vi "Extract_ROIs_miniScans.vi"(8 "error in (no error)":errorcluster, 10 "ROI Attributes":T1[](array[typedef]) {"ROI group ID" format="%#_6f"; "Laser Power (%)" format="%#_6f"; "Zoom" format="%#_6f"; "Frame Size" format="%#_6f"; "Number of lines" format="%#_6f"; "Composite ID" format="%#_6f"; "Angle (deg)" format="%#_6f"; "ROI Time (ns)" format="%#_6f"; "ROI ID" format="%#_6f"; "Pixels in ROI" format="%#_6f"; "ROI index" format="%#_6f"; "Z stop" format="%#_6f"; "Y stop" format="%#_6f"; "X stop" format="%#_6f"; "Z start" format="%#_6f"; "X start" format="%#_6f"; "Y start" format="%#_6f"}) -> (0 "error out":errorcluster, 1 "Total number of miniscans":i32, 2 "miniScan_Indices":dbl[](array[numeric]), 3 "ROI Coordinates (broken down to miniscans)":T2, 4 "Zoom":dbl[](array[numeric]), 5 "Number of pixels in single X miniscan":i32, 6 "number of rectangles":i32, 7 "number of POI":i32)   [LabVIEW 2017]
uses:
  Typedefs/ROI XY coordinates cluster.ctl
  User Interface/Visualisation/Functional Imaging Viewer/Typedefs/ROI parameters data type.ctl
panel:
  out "POI_Indices":dbl[](array[numeric])
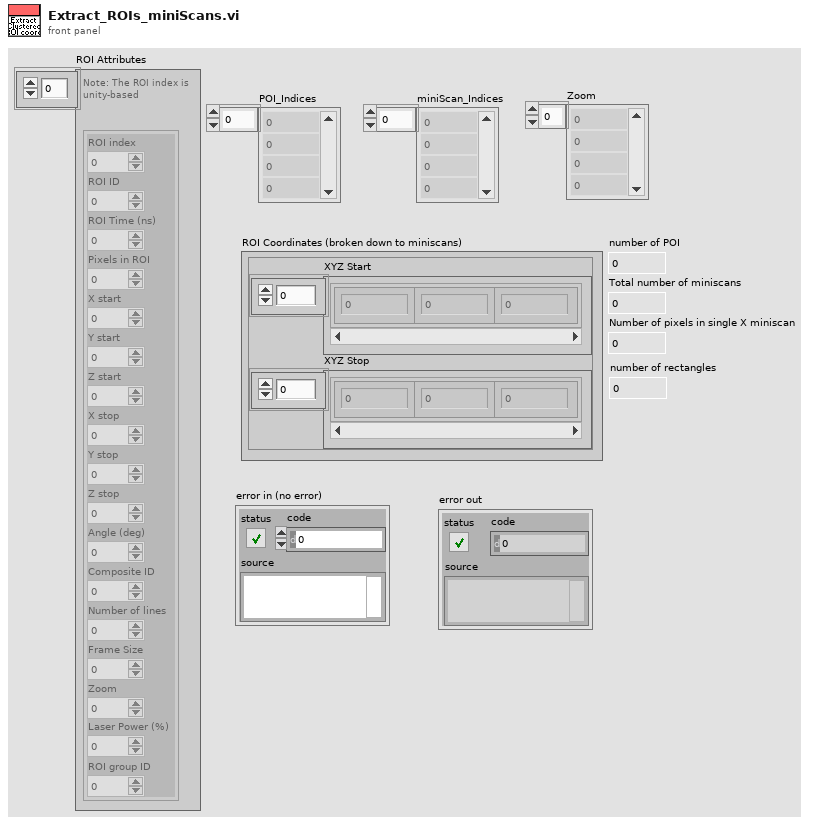
[diagram p1: front panel]
types:
  T1 = typedef "ROI parameters data type.ctl" = cluster{"ROI index":dbl, "ROI ID":dbl, "ROI Time (ns)":dbl, "Pixels in ROI":dbl, "X start":dbl, "Y start":dbl, "Z start":dbl, "X stop":dbl, "Y stop":dbl, "Z stop":dbl, "Angle (deg)":dbl, "Composite ID":dbl, "Number of lines":dbl, "Frame Size":dbl, "Zoom":dbl, "Laser Power (%)":dbl, "ROI group ID":dbl}
  T2 = typedef "ROI XY coordinates cluster.ctl" = cluster{"XYZ Start":cluster{"X":sgl, "Y":sgl, "Z":sgl}[], "XYZ Stop":cluster{"X":sgl, "Y":sgl, "Z":sgl}[]}
  T3 = cluster{"X start":dbl, "Y start":dbl, "Z start":dbl}[]
  T4 = cluster{"X start":dbl, "Y start":dbl, "Z start":dbl}
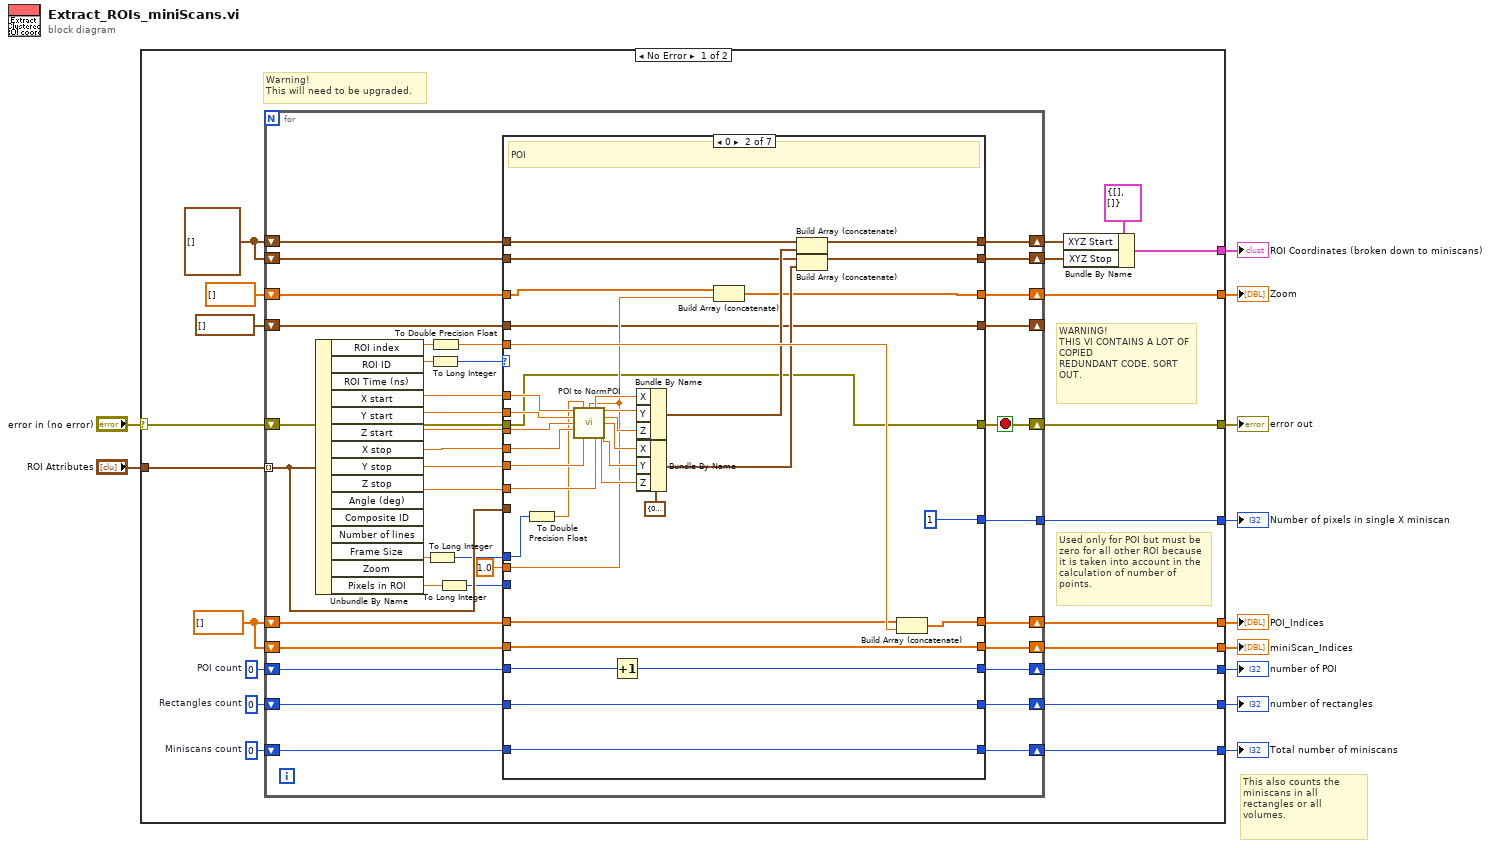
[diagram p0: block diagram]
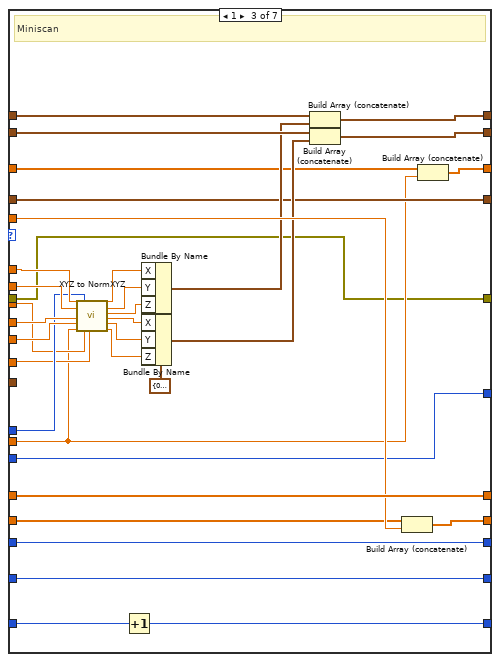
[diagram p3: hidden frame]
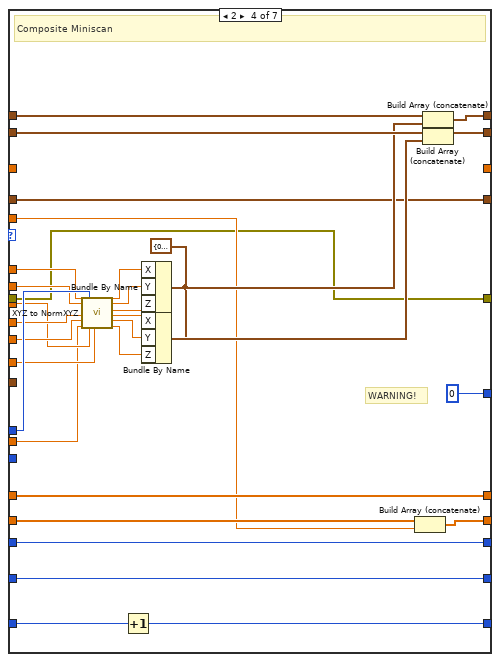
[diagram p4: hidden frame]
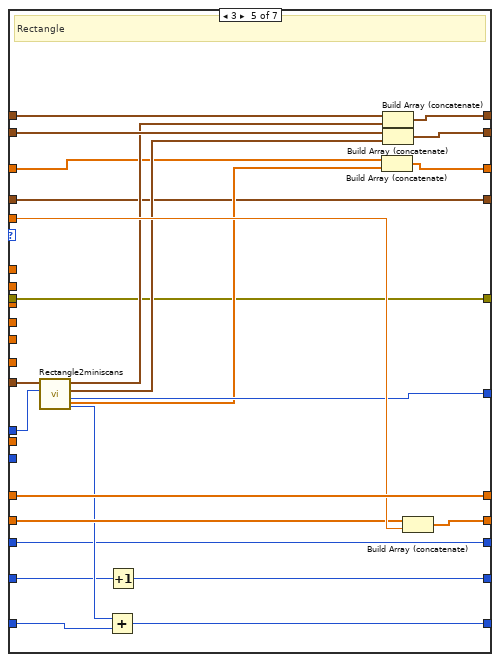
[diagram p5: hidden frame]
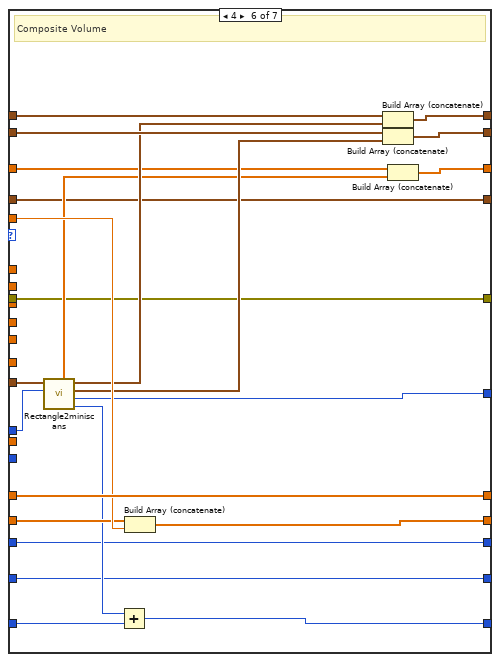
[diagram p6: hidden frame]
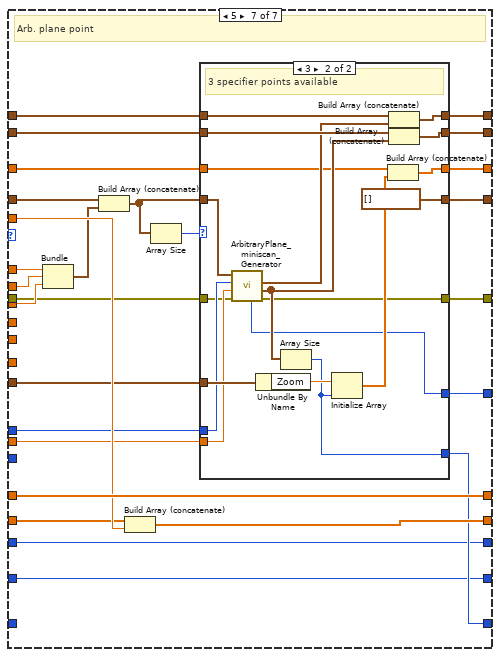
[diagram p7: hidden frame]
diagram:
  # "This also counts the miniscans in all rectangles or all volumes."
  n1 = case shown="No Error" "error in (no error)" {
    selector: "error in (no error)" -> [w15 w278]
    tunnel: [w14 w278] -> w10
    tunnel: [w23 _] -> w9
    tunnel: [w22 _] -> w8
    tunnel: [w21 _] -> w7
    tunnel: [w20 _] -> w6
    tunnel: [w19 _] -> w5
    tunnel: [w18 _] -> w4
    tunnel: [w17 _] -> w3
    tunnel: "ROI Attributes" -> [w16 _]
    tunnel: [w13 _] -> w1
    frame No Error {
      w12 = 0  # Rectangles count
      w25 = 0  # POI count
      w26 = 0  # Miniscans count
      w31 = cluster{"X":sgl, "Y":sgl, "Z":sgl}[] [] ("XYZ Coordinates")
      w32 = dbl[] []
      # "Used only for POI but must be zero for all other ROI because it is taken into account in the calculation of number of points."
      # "WARNING!\nTHIS VI CONTAINS A LOT OF COPIED \nREDUNDANT CODE. SORT OUT."
      # "Warning!\nThis will need to be upgraded."
      n2 = for {
        tunnel: w16 -> [w57] mode=indexing
        shift-right: [w67] -> w20
        shift-left: w32 -> [w66]
        shift-right: [w65] -> w19
        shift-left: w32 -> [w64]
        shift-right: [w63] -> w30
        shift-left: w31 -> [w62]
        shift-right: [w61] -> w29
        shift-left: w31 -> [w60]
        tunnel: [w56] -> w21
        shift-right: [w47] -> w22
        shift-left: dbl[] [] -> [w46]
        shift-right: [w42] -> w17
        shift-left: w26 -> [w43]
        shift-right: [w40] -> w18
        shift-left: w25 -> [w41]
        shift-right: [w39] -> _
        shift-left: T3 [] -> [w38]
        shift-right: [w36] -> w14
        shift-left: w15 -> [w37]
        shift-right: [w34] -> w13
        shift-left: w12 -> [w35]
        stop <- w36 stop-if-true
        n3 = Unbundle By Name(w57) -> ("ROI index"=w68:dbl, "ROI ID"=w69:dbl, "X start"=w53:dbl, "Y start"=w52:dbl, "Z start"=w51:dbl, "X stop"=w50:dbl, "Y stop"=w49:dbl, "Z stop"=w48:dbl, "Frame Size"=w55:dbl, "Pixels in ROI"=w45:dbl)  [unwired: 5 out]
        n4 = To Long Integer(number=w55) -> (32bit integer=w54:i32)
        n5 = To Long Integer(number=w69) -> (32bit integer=w58:i32)
        n6 = To Double Precision Float(number=w68) -> (double precision float=w59:dbl)
        n7 = To Long Integer(number=w45) -> (32bit integer=w44:i32)
        n8 = case shown="0" w58 {
          tunnel: w59 -> [_ w113 w146 w170 w202 w225 w252]
          tunnel: [w76 w112 w147 w179 w203 w226 w253] -> w67
          tunnel: w66 -> [w76 w111 w147 w179 w203 w226 w253]
          tunnel: [w75 w110 w145 w178 w201 w224 w251] -> w65
          tunnel: w64 -> [w75 w110 w144 w177 w200 w223 w250]
          tunnel: [w78 w89 w143 w176 w199 w222 w249] -> w63
          tunnel: w62 -> [w78 w82 w142 w175 w198 w221 w248]
          tunnel: [w77 w88 w141 w174 w197 w220 w247] -> w61
          tunnel: w60 -> [w77 w81 w140 w173 w196 w219 w246]
          tunnel: w57 -> [_ _ _ _ w195 w218 w234]
          tunnel: w54 -> [_ w106 w123 w169 w194 w215 w238]
          tunnel: [_ 1 ("No of Pixels") w134 0 ("No of Pixels in a single miniscan") w191 w214 w232] -> w56
          tunnel: w53 -> [_ w99 w127 w168 _ _ w243]
          tunnel: w52 -> [_ w98 w126 w167 _ _ w242]
          tunnel: w51 -> [_ w97 w120 w156 _ _ w241]
          tunnel: w50 -> [_ w96 w125 w166 _ _ _]
          tunnel: w49 -> [_ w95 w124 w165 _ _ _]
          tunnel: w48 -> [_ w94 w119 w155 _ _ _]
          tunnel: [_ w90 w136 _ w189 w212 w245] -> w47
          tunnel: w46 -> [_ w91 w135 _ w185 w211 w244]
          tunnel: [w70 w86 w114 w148 w180 w204 w227] -> w40
          tunnel: 1.0 ("Zoom") -> [_ w92 w117 w152 _ _ w231]
          tunnel: w44 -> [_ _ w134 _ _ _ _]
          tunnel: w43 -> [w74 w85 w122 w158 w187 w209 _]
          tunnel: [w74 w85 w121 w157 w186 w208 w233] -> w42
          tunnel: w41 -> [w70 w84 w114 w148 w180 w204 w227]
          tunnel: [w73 w83 w118 w153 w184 w207 w237] -> w39
          tunnel: w38 -> [w73 w83 w118 w153 w184 w207 w239]
          tunnel: w37 -> [w72 w80 w116 w150 w183 w206 w230]
          tunnel: [w72 w80 w116 w150 w183 w206 w229] -> w36
          tunnel: w35 -> [w71 w79 w115 w149 w182 w205 w228]
          tunnel: [w71 w79 w115 w149 w181 w205 w228] -> w34
          frame Default {
          }
          frame 0 {
            w109 = cluster{"X":dbl, "Y":dbl, "Z":dbl} {"X"=0.0, "Y"=0.0, "Z"=0.0} ("XYZ")
            # "POI"
            n9 = To Double Precision Float(number=w106) -> (double precision float=w93:dbl)
            n10 = call "POI to NormPOI.vi"("X start"=w99, "FrameSize"=w93, "Zoom"=w92, "Y start"=w98, "Z start"=w97, "X stop"=w96, "Y stop"=w95, "Z stop"=w94) -> ("Norm XStart"=w104:dbl, "Norm YStart"=w105:dbl, "Norm ZStart"=w103:dbl, "Norm XStop"=w102:dbl, "Norm YStop"=w101:dbl, "Norm ZStop"=w100:dbl)  [unwired: 2 in]
            n11 = Increment(x=w84) -> (x+1=w86:i32)
            n12 = Bundle By Name(cluster=w109, "X"=w104, "Y"=w105, "Z"=w103) -> (w108:cluster{"X":dbl, "Y":dbl, "Z":dbl})
            n13 = Bundle By Name(cluster=w109, "X"=w102, "Y"=w101, "Z"=w100) -> (w107:cluster{"X":dbl, "Y":dbl, "Z":dbl})
            n14 = Build Array (concatenate)(w91, w92) -> (w90:dbl[])
            n15 = Build Array (concatenate)(w82, w108) -> (w89:cluster{"X":dbl, "Y":dbl, "Z":dbl}[])
            n16 = Build Array (concatenate)(w81, w107) -> (w88:cluster{"X":dbl, "Y":dbl, "Z":dbl}[])
            n17 = Build Array (concatenate)(w111, w113) -> (w112:dbl[])
          }
          frame 1 {
            w139 = cluster{"X":dbl, "Y":dbl, "Z":dbl} {"X"=0.0, "Y"=0.0, "Z"=0.0} ("XYZ")
            # "Miniscan"
            n18 = call "XYZ to NormXYZ.vi"("X start"=w127, "Y start"=w126, "X stop"=w125, "Y stop"=w124, "Zoom (either ref or main zoom)"=w117, "FrameSize"=w123, "Z start"=w120, "Z stop"=w119) -> ("Norm X Start"=w133:dbl, "Norm Y Start"=w132:dbl, "Norm Z Start"=w131:dbl, "Norm X Stop"=w130:dbl, "Norm Y Stop"=w129:dbl, "Norm Z Stop"=w128:dbl)  [unwired: 6 in]
            n19 = Increment(x=w122) -> (x+1=w121:i32)
            n20 = Bundle By Name(cluster=w139, "X"=w133, "Y"=w132, "Z"=w131) -> (w138:cluster{"X":dbl, "Y":dbl, "Z":dbl})
            n21 = Bundle By Name(cluster=w139, "X"=w130, "Y"=w129, "Z"=w128) -> (w137:cluster{"X":dbl, "Y":dbl, "Z":dbl})
            n22 = Build Array (concatenate)(w142, w138) -> (w143:cluster{"X":dbl, "Y":dbl, "Z":dbl}[])
            n23 = Build Array (concatenate)(w140, w137) -> (w141:cluster{"X":dbl, "Y":dbl, "Z":dbl}[])
            n24 = Build Array (concatenate)(w144, w146) -> (w145:dbl[])
            n25 = Build Array (concatenate)(w135, w117) -> (w136:dbl[])
          }
          frame 2 {
            w151 = cluster{"X":dbl, "Y":dbl, "Z":dbl} {"X"=0.0, "Y"=0.0, "Z"=0.0} ("XYZ")
            # "WARNING!"
            # "Composite Miniscan"
            n26 = call "XYZ to NormXYZ.vi"("X start"=w168, "Y start"=w167, "X stop"=w166, "Y stop"=w165, "Zoom (either ref or main zoom)"=w152, "FrameSize"=w169, "Z start"=w156, "Z stop"=w155) -> ("Norm X Start"=w164:dbl, "Norm Y Start"=w163:dbl, "Norm Z Start"=w162:dbl, "Norm X Stop"=w161:dbl, "Norm Y Stop"=w160:dbl, "Norm Z Stop"=w159:dbl)  [unwired: 6 in]
            n27 = Increment(x=w158) -> (x+1=w157:i32)
            n28 = Bundle By Name(cluster=w151, "X"=w164, "Y"=w163, "Z"=w162) -> (w172:cluster{"X":dbl, "Y":dbl, "Z":dbl})
            n29 = Bundle By Name(cluster=w151, "X"=w161, "Y"=w160, "Z"=w159) -> (w171:cluster{"X":dbl, "Y":dbl, "Z":dbl})
            n30 = Build Array (concatenate)(w177, w170) -> (w178:dbl[])
            n31 = Build Array (concatenate)(w175, w172) -> (w176:cluster{"X":dbl, "Y":dbl, "Z":dbl}[])
            n32 = Build Array (concatenate)(w173, w171) -> (w174:cluster{"X":dbl, "Y":dbl, "Z":dbl}[])
          }
          frame 3 {
            # "Rectangle"
            n33 = call "Rectangle2miniscans.vi"("Frame Size"=w194, "X-Y-Z coordinates"=w195) -> ("No of Miniscans"=w188:i32, "No of Pixels in a single miniscan"=w191:i32, "XYZ Stop"=w192:cluster{"X":dbl, "Y":dbl, "Z":dbl}[], "XYZ Start"=w193:cluster{"X":dbl, "Y":dbl, "Z":dbl}[], "Zoom"=w190:dbl[])  [unwired: 5 in]
            n34 = Add(x=w188, y=w187) -> (x+y=w186:i32)
            n35 = Increment(x=w182) -> (x+1=w181:i32)
            n36 = Build Array (concatenate)(w185, w190) -> (w189:dbl[])
            n37 = Build Array (concatenate)(w198, w193) -> (w199:cluster{"X":dbl, "Y":dbl, "Z":dbl}[])
            n38 = Build Array (concatenate)(w196, w192) -> (w197:cluster{"X":dbl, "Y":dbl, "Z":dbl}[])
            n39 = Build Array (concatenate)(w200, w202) -> (w201:dbl[])
          }
          frame 4 {
            # "Composite Volume"
            n40 = call "Rectangle2miniscans.vi"("Frame Size"=w215, "X-Y-Z coordinates"=w218) -> ("No of Miniscans"=w210:i32, "No of Pixels in a single miniscan"=w214:i32, "XYZ Stop"=w216:cluster{"X":dbl, "Y":dbl, "Z":dbl}[], "XYZ Start"=w217:cluster{"X":dbl, "Y":dbl, "Z":dbl}[], "Zoom"=w213:dbl[])  [unwired: 5 in]
            n41 = Add(x=w210, y=w209) -> (x+y=w208:i32)
            n42 = Build Array (concatenate)(w223, w225) -> (w224:dbl[])
            n43 = Build Array (concatenate)(w221, w217) -> (w222:cluster{"X":dbl, "Y":dbl, "Z":dbl}[])
            n44 = Build Array (concatenate)(w219, w216) -> (w220:cluster{"X":dbl, "Y":dbl, "Z":dbl}[])
            n45 = Build Array (concatenate)(w211, w213) -> (w212:dbl[])
          }
          frame 5 {
            # "Arb. plane point"
            n46 = Bundle("X start"=w243, "Y start"=w242, "Z start"=w241) -> (w240:T4)  [unwired: 1 in]
            n47 = Build Array (concatenate)(w239, w240) -> (w236:T3)
            n48 = Build Array (concatenate)(w250, w252) -> (w251:dbl[])
            n49 = Array Size(array=w236) -> (size(s)=w235:i32)
            n50 = case shown="3" w235 {
              tunnel: [w257 w277] -> w249
              tunnel: w248 -> [w257 w276]
              tunnel: [w256 w275] -> w247
              tunnel: w246 -> [w256 w274]
              tunnel: [w255 w273] -> w245
              tunnel: w244 -> [w255 w264]
              tunnel: w236 -> [w258 w272]
              tunnel: w238 -> [_ w263]
              tunnel: [w258 T3 []] -> w237
              tunnel: w234 -> [_ w269]
              tunnel: [_ w265] -> w233
              tunnel: [_ w260] -> w232
              tunnel: w231 -> [_ w262]
              tunnel: w230 -> [w254 w261]
              tunnel: [w254 w259] -> w229
              frame Default {
                # "< than 3 specifier points"
              }
              frame 3 {
                # "3 specifier points available"
                n51 = call "ArbitraryPlane_miniscan_Generator.vi"("error in"=w261, "Main Zoom"=w262, "Frame Size"=w263, "Input data"=w272) -> ("error out"=w259:errorcluster, "XYZ Stop Norm"=w268:cluster{"X":sgl, "Y":sgl, "Z":sgl}[], "XYZ Start Norm"=w270:cluster{"X":sgl, "Y":sgl, "Z":sgl}[], "Number of pixels in single X miniscan"=w260:i32)  [unwired: 3 in, 1 out]
                n52 = Unbundle By Name(w269) -> ("Zoom"=w267:dbl)
                n53 = Array Size(array=w268) -> (size(s)=w265:i32)
                n54 = Initialize Array(w267, w265) -> (w266:dbl[])
                n55 = Build Array (concatenate)(w264, w266) -> (w273:dbl[])
                n56 = Build Array (concatenate)(w276, w270) -> (w277:cluster{"X":dbl, "Y":dbl, "Z":dbl}[])
                n57 = Build Array (concatenate)(w274, w268) -> (w275:cluster{"X":dbl, "Y":dbl, "Z":dbl}[])
              }
            }
          }
        }
      }
      n58 = Bundle By Name(cluster=T2 {"XYZ Start"=[], "XYZ Stop"=[]} ("ROI Coordinates"), "XYZ Start"=w30, "XYZ Stop"=w29) -> (w23:T2)
    }
    frame Error {
    }
  }
  "error out" <- w10
  "ROI Coordinates (broken down to miniscans)" <- w9
  "POI_Indices" <- w6
  "miniScan_Indices" <- w5
  "Total number of miniscans" <- w3
  "Number of pixels in single X miniscan" <- w7
  "Zoom" <- w8
  "number of POI" <- w4
  "number of rectangles" <- w1
